vi "Load_Analogue_Data_2_Time_traces_1D.vi"(2 "Ch Index":i32, 3 "Voltage Array":dbl[](array[numeric]), 4 "Sampling Rate (Hz)":dbl) -> ()   [LabVIEW 2017]
uses:
  Globals/Meas_global.vi
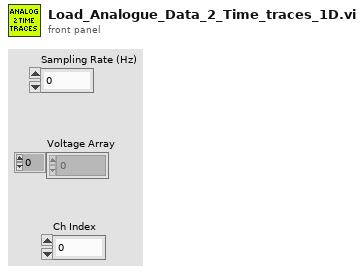
[diagram p1: front panel]
types:
  T1 = typedef "Analysis_info_cluster.ctl" = cluster{"Colour":u32, "Inst type":T2, "Inst name":string, "Symbol":string, "Code name":string, "Extra Info":string, "Inst Array":T3, "Extra Titles":string[], "Extra Values":string[], "U":dbl, "u^2":dbl, "u^3":dbl, "u^4":dbl, "Skew_u":dbl, "Kurt_u":dbl, "Sd Error in Mean":dbl, "% u'/U":dbl, "X":dbl, "Y":dbl, "Z":dbl, "Timescale integral Estimate":dbl, "Sd Error in Variance":dbl, "Calib File":path, "Calib Constants":dbl[], "Output Position":bool, "Full Stats":bool, "Av Sampling Rate":dbl, "Av No of Samples":dbl, "Total Meas Time (s)":dbl, "ADAM Ch Name":string, "Max value":dbl, "Min value":dbl, "Sync Delay Time (s)":dbl, "Device ID":string, "Req Sample Rate Hz":dbl}
  T2 = typedef "Inst_type.ctl" = enum16{"Propeller anemometer", "Raw voltage", "Pressure Transducer", "Pitot-static tube", "Preston tube", "Hot wire", "Cross wire 1", "Cross wire 2", "Generic Linear", "Generic Polynomial", "Generic BackPoly", "Fast FID", "Thermocouple", "Cold wire", "Pulsed Wire", "LDA Vel", "LDA Tran time", "LDA Arr time", "Microphone"}
  T3 = typedef "Instrument_Array.ctl" = enum16{"PWA", "LDA", "Analogue"}
  T4 = typedef "Time_Trace_Cluster.ctl" = cluster{"Weighting":dbl[], "Time (s)":dbl[], "Voltage":dbl[], "Eng Values":dbl[]}
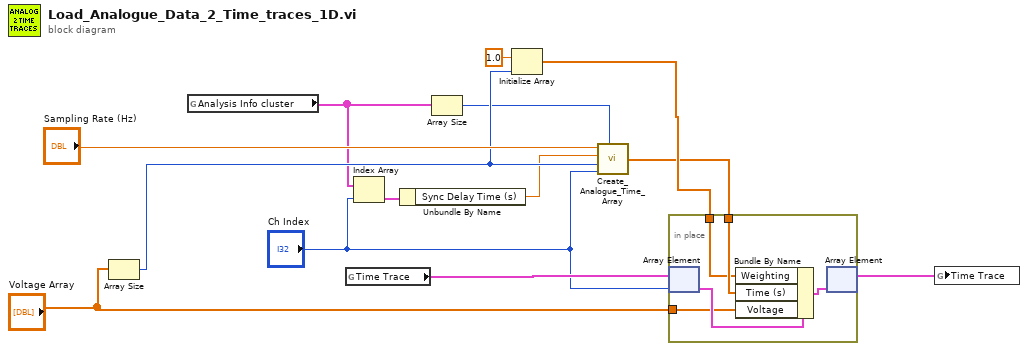
[diagram p0: block diagram]
diagram:
  n1 = Array Size(array="Voltage Array") -> (size(s)=w7:i32)
  n2 = global read "Meas_global.vi" "Analysis Info cluster"() -> (w4:T1[])
  n3 = global read "Meas_global.vi" "Time Trace"() -> (w5:T4[])
  n4 = Index Array(array=w4, index="Ch Index") -> (element=w2:T1)
  n5 = Unbundle By Name(w2) -> ("Sync Delay Time (s)"=w1:dbl)
  n6 = Array Size(array=w4) -> (size(s)=w6:i32)
  n7 = Initialize Array(1.0 ("element"), w7) -> (w13:dbl[])
  n8 = call "Create_Analogue_Time_Array.vi"("Sampling Rate (Hz)"="Sampling Rate (Hz)", "Sync Delay (s)"=w1, "No of Samples"=w7, "Index"="Ch Index", "No Of Analogue Chs"=w6) -> ("Times"=w8:dbl[])
  n9 = in-place {
    in-place-border: "Voltage Array" -> [w17]
    in-place-border: w8 -> [w15]
    in-place-border: w13 -> [w14]
    n10 = in-place-array #1(w5, "Ch Index") -> (w18:T4)
    n11 = Bundle By Name(cluster=w18, "Weighting"=w14, "Time (s)"=w15, "Voltage"=w17) -> (w16:T4)
    n12 = in-place-array #1(w16) -> (w11:T4[])  [unwired: 1 out]
  }
  n13 = global write "Meas_global.vi" "Time Trace"(w11) -> ()
